vi "Priority Dequeue.vi"(8 "error in (no error)":errorcluster, 9 "Timeout mS (-1)":i32=-1, 11 "Priority Message Queue in":refnum<class "Priority Message Queue.lvclass">) -> (0 "error out":errorcluster, 1 "Timed Out":bool, 2 "Message":refnum<class "Message.lvclass">, 3 "Priority Message Queue out":refnum<class "Priority Message Queue.lvclass">, 4 "Priority":i32)   [LabVIEW 2020, in "Artifex.lvlib" / "Priority Message Queue.lvclass"]
uses:
  Priority Message Queue.lvclass
  Message/Message.lvclass
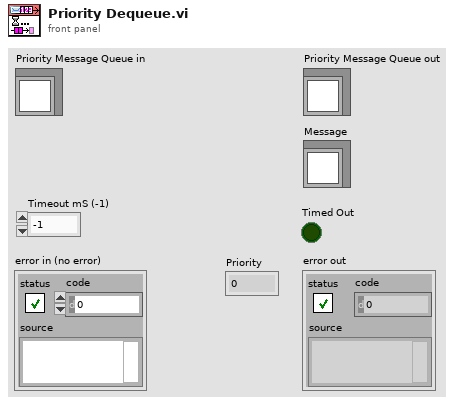
[diagram p1: front panel]
types:
  T1 = typedef "Artifex.lvlib/Priority Message Queue.lvclass/Ref Data.ctl" = cluster{"# Waiting":u32, "Buffers":refnum<queue>[], "Wait Msg":refnum<queue>, "Wait Prior":refnum<queue>}
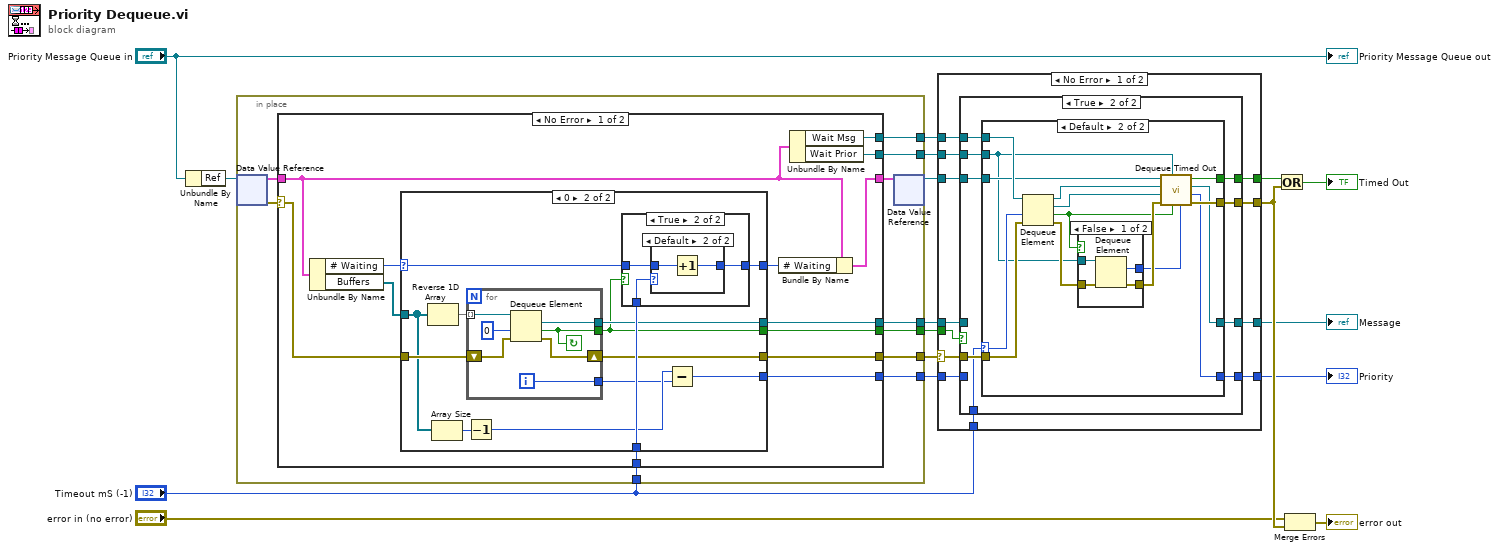
[diagram p0: block diagram]
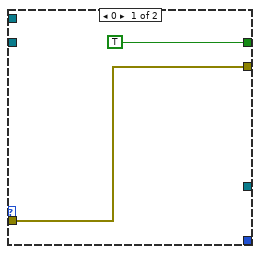
[diagram p3: hidden frame]
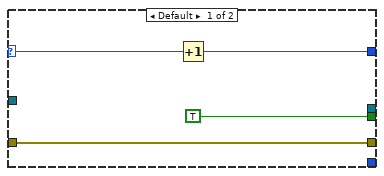
[diagram p6: hidden frame]
diagram:
  n1 = Unbundle By Name("Priority Message Queue in") -> ("Ref"=w14:refnum<data-value>)
  n2 = in-place {
    in-place-border: "Timeout mS (-1)" -> [w24]
    in-place-border: [w23] -> w8
    in-place-border: [w22] -> w9
    in-place-border: [w21] -> w10
    in-place-border: [w20] -> w11
    in-place-border: [w19] -> w12
    in-place-border: [w18] -> w13
    n3 = in-place-dvr #1(w14) -> (w26:T1, w27:errorcluster)
    n4 = case shown="No Error" w27 {
      selector: w27 -> [w36 w72]
      tunnel: w26 -> [w34 w73]
      tunnel: [w40 w73] -> w25
      tunnel: w24 -> [w35 _]
      tunnel: [w33 _] -> w23
      tunnel: [w32 _] -> w22
      tunnel: [w31 _] -> w21
      tunnel: [w30 _] -> w20
      tunnel: [w29 _] -> w19
      tunnel: [w28 w72] -> w18
      frame No Error {
        n5 = Unbundle By Name(w34) -> ("# Waiting"=w39:u32, "Buffers"=w38:refnum<queue>[])
        n6 = case shown="0" w39 {
          selector: w39 -> [w44 w55]
          tunnel: w38 -> [_ w50]
          tunnel: [w43 w54] -> w37
          tunnel: w36 -> [w41 w56]
          tunnel: w35 -> [_ w53]
          tunnel: [_ w52] -> w31
          tunnel: [TRUE ("timed out?") w51] -> w30
          tunnel: [w41 w46] -> w28
          tunnel: [_ w45] -> w29
          frame Default {
            n7 = Increment(x=w44) -> (x+1=w43:u32)
          }
          frame 0 {
            n8 = Reverse 1D Array(array=w50) -> (reversed array=w57:refnum<queue>[])
            n9 = Array Size(array=w50) -> (size(s)=w49:i32)
            n10 = Decrement(x=w49) -> (x-1=w48:i32)
            n11 = for {
              tunnel: w57 -> [w71] mode=indexing
              shift-right: [w68] -> w46
              shift-left: w56 -> [w69]
              tunnel: [w66] -> w51
              tunnel: [w67] -> w52
              tunnel: [w65] -> w47
              i -> [w65]
              stop <- w66 continue-if-true
              n12 = Dequeue Element(queue=w71, timeout in ms (-1)=0, error in (no error)=w69) -> (element=w67:refnum<class "Message.lvclass">, timed out?=w66:bool, error out=w68:errorcluster)  [unwired: 1 out]
            }
            n13 = case shown="True" w51 {
              tunnel: w55 -> [w58 w60]
              tunnel: [w58 w59] -> w54
              tunnel: w53 -> [_ w61]
              frame False {
              }
              frame True {
                n14 = case shown="Default" w61 {
                  tunnel: w60 -> [w62 w64]
                  tunnel: [w62 w63] -> w59
                  frame 0 {
                  }
                  frame Default {
                    n15 = Increment(x=w64) -> (x+1=w63:u32)
                  }
                }
              }
            }
            n16 = Subtract(x=w48, y=w47) -> (x-y=w45:i32)
          }
        }
        n17 = Bundle By Name(cluster=w34, "# Waiting"=w37) -> (w40:T1)
        n18 = Unbundle By Name(w34) -> ("Wait Msg"=w33:refnum<queue>, "Wait Prior"=w32:refnum<queue>)
      }
      frame Error {
      }
    }
    n19 = in-place-dvr #1(w25) -> (w2:refnum<data-value>)  [unwired: 1 out]
  }
  n20 = case shown="No Error" w13 {
    selector: w13 -> [w77 w122]
    tunnel: w12 -> [w81 w121]
    tunnel: w11 -> [w85 _]
    tunnel: w10 -> [w82 w120]
    tunnel: w9 -> [w83 _]
    tunnel: w8 -> [w84 _]
    tunnel: [w76 w122] -> w17
    tunnel: [w74 w121] -> w6
    tunnel: [w75 w120] -> w5
    tunnel: "Timeout mS (-1)" -> [w80 _]
    tunnel: [w79 _] -> w3
    tunnel: w2 -> [w78 _]
    frame No Error {
      n21 = case shown="True" w85 {
        tunnel: w84 -> [_ w94]
        tunnel: w83 -> [_ w92]
        tunnel: w82 -> [w86 _]
        tunnel: w81 -> [w87 _]
        tunnel: w80 -> [_ w96]
        tunnel: [_ w95] -> w79
        tunnel: w78 -> [_ w93]
        tunnel: w77 -> [w88 w97]
        tunnel: [w88 w91] -> w76
        tunnel: [w86 w90] -> w75
        tunnel: [w87 w89] -> w74
        frame False {
        }
        frame True {
          n22 = case shown="Default" w96 {
            selector: w96 -> [_ w113]
            tunnel: [TRUE w110] -> w95
            tunnel: w94 -> [_ w112]
            tunnel: w93 -> [_ w111]
            tunnel: w92 -> [_ w104]
            tunnel: w97 -> [w98 w109]
            tunnel: [w98 w102] -> w91
            tunnel: [_ w101] -> w90
            tunnel: [_ w100] -> w89
            frame 0 {
            }
            frame Default {
              n23 = Dequeue Element(queue=w112, timeout in ms (-1)=w113, error in (no error)=w109) -> (queue out=w107:refnum<queue>, element=w108:refnum<class "Message.lvclass">, timed out?=w105:bool, error out=w106:errorcluster)
              n24 = case shown="False" w105 {
                tunnel: w106 -> [w117 w119]
                tunnel: w104 -> [w118 _]
                tunnel: [w116 _] -> w103
                tunnel: [w115 w119] -> w114
                frame False {
                  n25 = Dequeue Element(queue=w118, error in (no error)=w117) -> (element=w116:i32, error out=w115:errorcluster)  [unwired: 1 in, 2 out]
                }
                frame True {
                }
              }
              n26 = call "Dequeue Timed Out.vi"("Priority In"=w103, "Timed Out"=w105, "Wait Prior"=w104, "error in (no error)"=w114, "Message In"=w108, "Wait Msg"=w107, "Ref"=w111) -> ("error out"=w102:errorcluster, "Priority"=w100:i32, "Message"=w101:refnum<class "Message.lvclass">, "Really Timed Out"=w110:bool)  [unwired: 1 in]
            }
          }
        }
      }
    }
    frame Error {
    }
  }
  "Message" <- w5
  "Priority" <- w6
  n27 = Or(x=w3, y=w17) -> (x .or. y?=→"Timed Out":bool)
  n28 = Merge Errors("error in (no error)", w17) -> (→"error out":errorcluster)
  "Priority Message Queue out" <- "Priority Message Queue in"
